vi "Clear out and err indicators.vi"(8 "error in (no error)":errorcluster, 11 "Kasli Wrapper 2.0 in":refnum<class "Kasli Wrapper 2.0.lvclass">) -> (0 "error out":errorcluster, 3 "Kasli Wrapper 2.0 out":refnum<class "Kasli Wrapper 2.0.lvclass">)   [LabVIEW 2020, in "Kasli Wrapper 2.0.lvlib" / "Kasli Wrapper 2.0.lvclass"]
uses:
  Kasli Wrapper 2.0.lvclass
  TALOS/TALOS_PPL.lvlibp/Father of all uServices/Father of all uServices/Father of all uServices.lvclass
  C:/Users/aegis/Documents/CIRCUS/TALOS/TALOS_PPL.lvlibp/Father of all uServices/Father of all uServices/Father of all uServices.lvclass
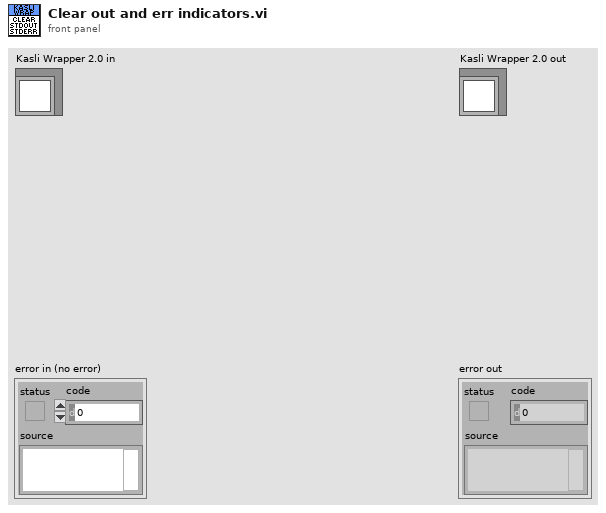
[diagram p1: front panel]
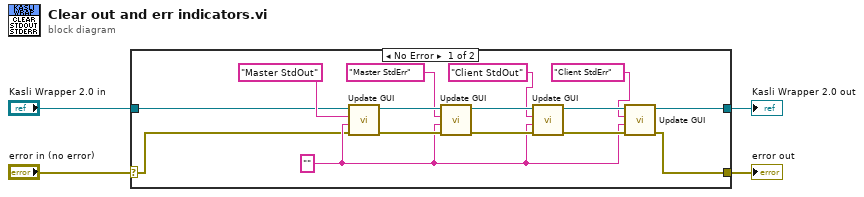
[diagram p0: block diagram]
diagram:
  n1 = case shown="No Error" "error in (no error)" {
    selector: "error in (no error)" -> [w6 w21]
    tunnel: [w5 w21] -> w3
    tunnel: [w7 w20] -> w1
    tunnel: "Kasli Wrapper 2.0 in" -> [w8 w20]
    frame No Error {
      w13 = ""
      n2 = call "Update GUI.vi"("error in (no error)"=w6, "Data"=w13, "GUI Item Name"="Master StdOut", "uService Template in"=w8) -> ("error out"=w16:errorcluster, "uService Template out"=w19:refnum<class "Kasli Wrapper 2.0.lvclass">)  [unwired: 6 in]
      n3 = call "Update GUI.vi"("error in (no error)"=w16, "Data"=w13, "GUI Item Name"="Master StdErr", "uService Template in"=w19) -> ("error out"=w15:errorcluster, "uService Template out"=w18:refnum<class "Kasli Wrapper 2.0.lvclass">)  [unwired: 6 in]
      n4 = call "Update GUI.vi"("error in (no error)"=w15, "Data"=w13, "GUI Item Name"="Client StdOut", "uService Template in"=w18) -> ("error out"=w14:errorcluster, "uService Template out"=w17:refnum<class "Kasli Wrapper 2.0.lvclass">)  [unwired: 6 in]
      n5 = call "Update GUI.vi"("error in (no error)"=w14, "Data"=w13, "GUI Item Name"="Client StdErr", "uService Template in"=w17) -> ("error out"=w5:errorcluster, "uService Template out"=w7:refnum<class "Kasli Wrapper 2.0.lvclass">)  [unwired: 6 in]
    }
    frame Error {
    }
  }
  "error out" <- w3
  "Kasli Wrapper 2.0 out" <- w1
